vi "Top Level State Machine - Framework Only (working without scripting VIs).vi"() -> ()   [LabVIEW 2014]
uses:
  Scripting States.ctl
  System.Windows.Forms
panel:
  out "Elapsed Time":dbl format="%<%H:%M:%S>t"
  in  "ProgressBar":refnum<k24>(container)
  out "Progress Bar 2":u8
  in  "?":T1
  out "Status Log":string
  out "Progress Bar":u8(slide) scale=0.0..9.0
  # "#TestingOnly"
  # "Append string with new steps as they're reached\nAppend error with source information (including current state) to end if it occurs"
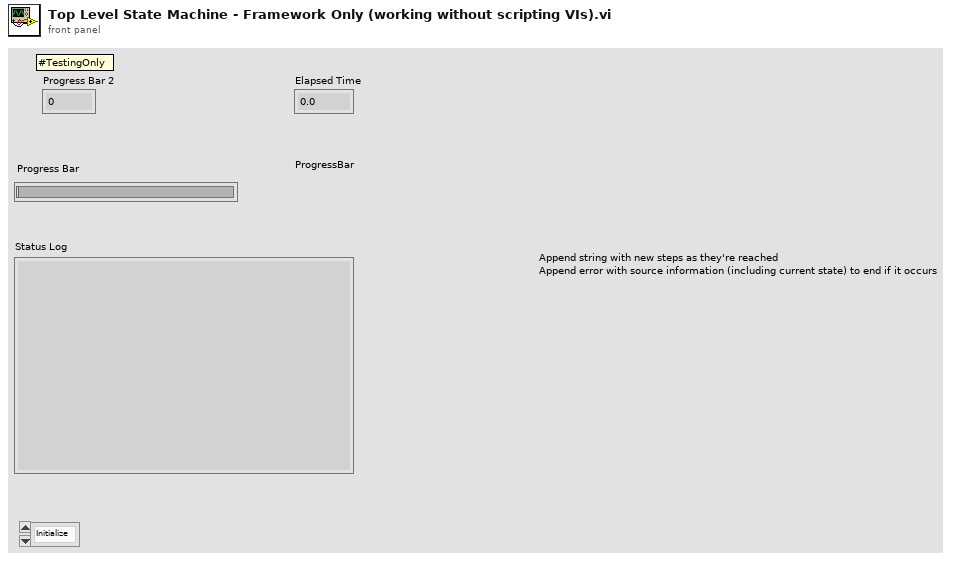
[diagram p1: front panel]
types:
  T1 = typedef "Scripting States.ctl" = enum16{"Initialize", "Modify Dequeue Commands", "Modify Enqueue Data", "Create Project FIFOs", "Populate FIFO Names in Engine", "Create and Place IO Nodes", "Place SPI Engine", "Modify I/O Pin Names", "Modify I/O Pin Enable", "End"}
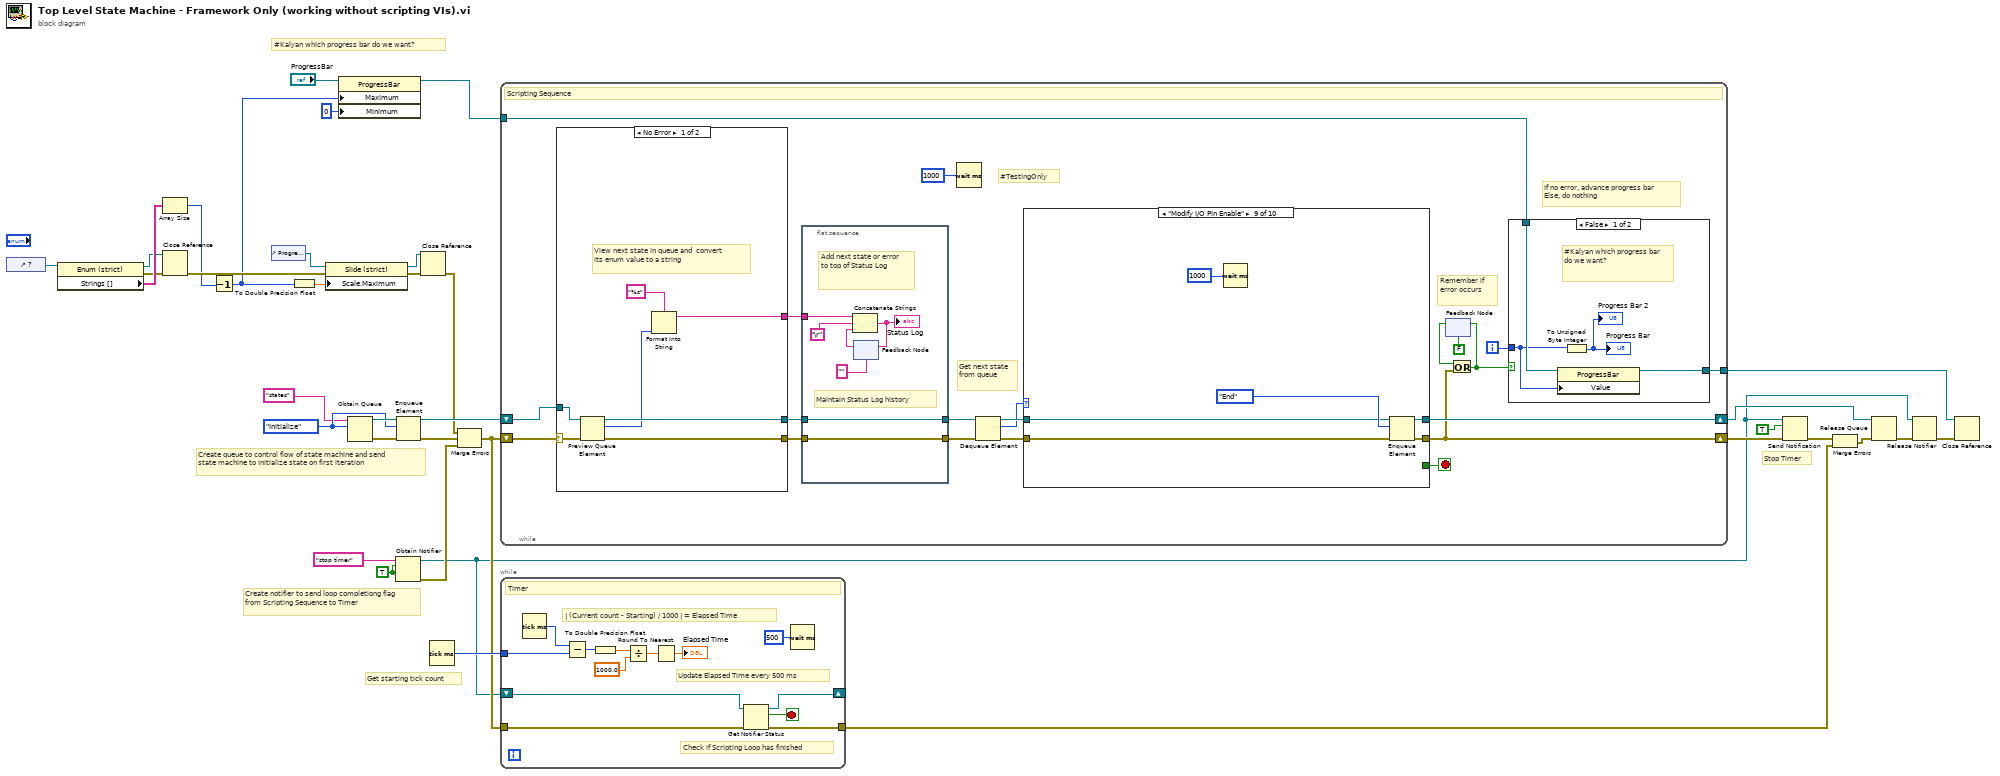
[diagram p0: block diagram]
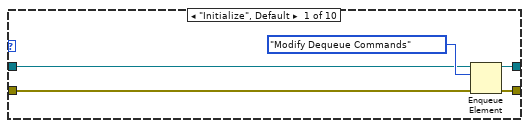
[diagram p3: hidden frame]
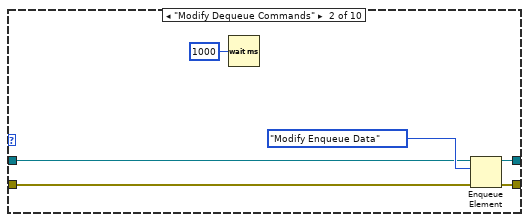
[diagram p4: hidden frame]
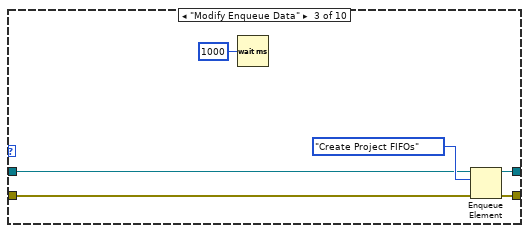
[diagram p5: hidden frame]
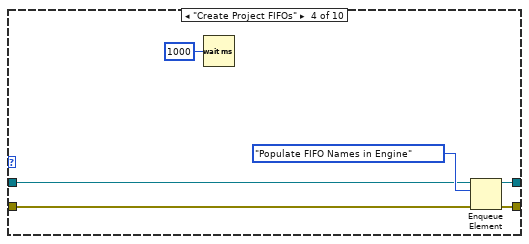
[diagram p6: hidden frame]
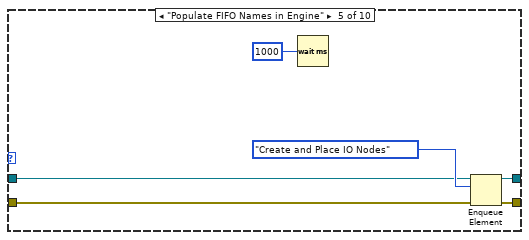
[diagram p7: hidden frame]
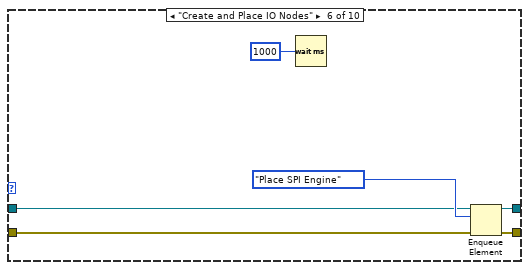
[diagram p8: hidden frame]
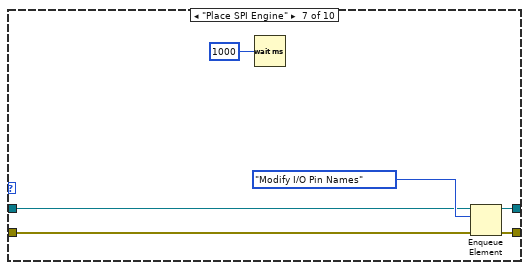
[diagram p9: hidden frame]
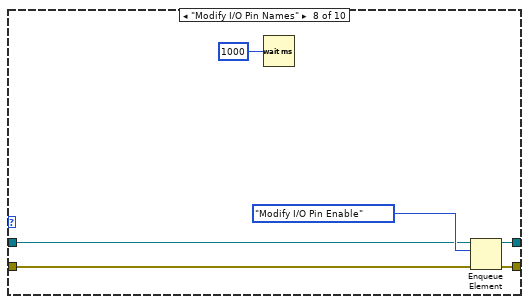
[diagram p10: hidden frame]
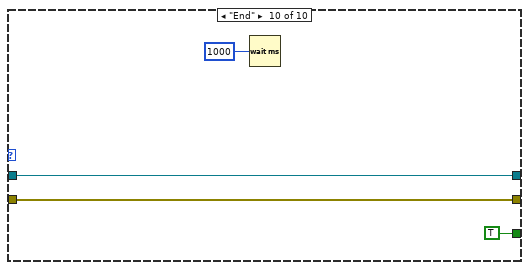
[diagram p11: hidden frame]
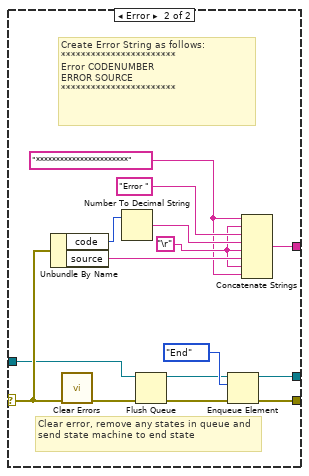
[diagram p12: hidden frame]
diagram:
  w13 = TRUE ("create if not found? (T)")
  w30 = Scripting_States."Initialize"
  # "Get starting tick count"
  # "Stop Timer"
  # "Create notifier to send loop completiong flag from Scripting Sequence to Timer"
  # "Create queue to control flow of state machine and send state machine to Initialize state on first iteration"
  # "#Kalyan which progress bar do we want?"
  n1 = control-ref of="?"() -> (w36:refnum<vi>)
  n2 = property on="Property Node" class="Enum (strict)"(reference=w36) -> (reference out=w23:refnum<vi>, error out=w24:errorcluster, "Strings []"=w35:string[])  [unwired: 1 in]
  n3 = Array Size(array=w35) -> (size(s)=w20:i32)
  n4 = Close Reference(reference=w23, error in (no error)=w24) -> (error out=w21:errorcluster)
  n5 = Decrement(x=w20) -> (x-1=w18:i32)
  n6 = control-ref of="Progress Bar"() -> (w34:refnum<vi>)
  n7 = To Double Precision Float(number=w18) -> (double precision float=w33:dbl)
  n8 = property on="Property Node" class="Slide (strict)"(reference=w34, error in=w21, "Scale.Maximum"=w33) -> (reference out=w25:refnum<vi>, error out=w26:errorcluster)
  n9 = property class="ProgressBar"(reference="ProgressBar", "Maximum"=w18, "Minimum"=0) -> (reference out=w8:refnum<k24>)  [unwired: 1 in, 1 out]
  n10 = Obtain Queue(name (unnamed)="states", element data type=w30) -> (queue out=w31:refnum<queue>, error out=w32:errorcluster)  [unwired: 3 in, 1 out]
  n11 = Obtain Notifier(name (unnamed)="stop timer", notification data type=w13, create if not found? (T)=w13) -> (notifier out=w1:refnum<notifier>, error out=w15:errorcluster)  [unwired: 1 in, 1 out]
  n12 = Enqueue Element(queue=w31, element=w30, error in (no error)=w32) -> (queue out=w28:refnum<queue>, error out=w27:errorcluster)  [unwired: 1 in, 1 out]
  n13 = Close Reference(reference=w25, error in (no error)=w26) -> (error out=w22:errorcluster)
  n14 = Tick Count (ms)() -> (millisecond timer value=w16:u32)
  n15 = Merge Errors(w22, w27, w15) -> (w14:errorcluster)
  n16 = while {
    shift-right: [w48] -> w3
    shift-left: w14 -> [w56]
    shift-right: [w50] -> w2
    shift-left: w28 -> [w55]
    tunnel: [w38] -> w9
    tunnel: w8 -> [w37]
    i -> [w49]
    stop <- w51 stop-if-true
    # "If no error, advance progress bar\nElse, do nothing"
    # "Remember if error occurs"
    # "Get next state from queue"
    # "#TestingOnly"
    # "Scripting Sequence"
    n17 = case shown="No Error" w56 {
      selector: w56 -> [w132 w142]
      tunnel: [w126 w144] -> w43
      tunnel: w55 -> [w131 w137]
      tunnel: [w129 w141] -> w42
      tunnel: [w130 w140] -> w40
      frame No Error {
        # "View next state in queue and  convert its enum value to a string"
        n18 = Preview Queue Element(queue=w131, error in (no error)=w132) -> (queue out=w130:refnum<queue>, element=w127:T1, error out=w129:errorcluster)  [unwired: 1 in, 1 out]
        n19 = Format Into String "Format Into String"(format string="%s", w127) -> (resulting string=w126:string)  [unwired: 2 in, 1 out]
      }
      frame Error {
        w133 = "***********************" ("string")
        w134 = "\r"
        # "Create Error String as follows:\n***********************\nError CODENUMBER\nERROR SOURCE\n***********************"
        # "Clear error, remove any states in queue and send state machine to end state"
        n20 = Unbundle By Name(w142) -> ("code"=w145:i32, "source"=w147:string)
        n21 = call <vilib>:"Clear Errors.vi"("error in (no error)"=w142) -> ("error out"=w139:errorcluster)  [unwired: 5 in, 1 out]
        n22 = Number To Decimal String(number=w145) -> (decimal integer string=w146:string)  [unwired: 1 in]
        n23 = Flush Queue(queue=w137, error in (no error)=w139) -> (queue out=w136:refnum<queue>, error out=w138:errorcluster)  [unwired: 1 out]
        n24 = Enqueue Element(queue=w136, element=Scripting_States."End", error in (no error)=w138) -> (queue out=w140:refnum<queue>, error out=w141:errorcluster)  [unwired: 1 in, 1 out]
        n25 = Concatenate Strings(w133, w134, "Error " ("string"), w146, w134, w147, w134, w133) -> (w144:string)
      }
    }
    n26 = flat-sequence {
      tunnel: w43 -> [w59]
      tunnel: w42 -> [w58]
      tunnel: [w58] -> w41
      tunnel: [w57] -> w39
      tunnel: w40 -> [w57]
      frame #0 {
        # "Maintain Status Log history"
        # "Add next state or error to top of Status Log"
        n27 = feedback #1("") -> (w61:string)
        n28 = Concatenate Strings(w59, "\r", w61) -> (w62:string)
        "Status Log" <- w62
        n29 = feedback-in #1(w62) -> ()
      }
    }
    n30 = Wait (ms)(milliseconds to wait=u32 1000) -> ()  [unwired: 1 out]
    n31 = Dequeue Element(queue=w39, error in (no error)=w41) -> (queue out=w53:refnum<queue>, element=w52:T1, error out=w54:errorcluster)  [unwired: 1 in, 1 out]
    n32 = case shown="\"Modify I/O Pin Enable\"" w52 {
      tunnel: [w72 w78 w84 w90 w96 w102 w108 w114 w120 w122] -> w48
      tunnel: [w73 w79 w85 w91 w97 w103 w109 w115 w121 w124] -> w50
      tunnel: [_ _ _ _ _ _ _ _ _ TRUE] -> w51
      tunnel: w54 -> [w70 w75 w81 w86 w93 w99 w105 w111 w117 w122]
      tunnel: w53 -> [w69 w76 w82 w88 w94 w100 w106 w112 w118 w124]
      frame "Initialize", Default {
        n33 = Enqueue Element(queue=w69, element=Scripting_States."Modify Dequeue Commands", error in (no error)=w70) -> (queue out=w73:refnum<queue>, error out=w72:errorcluster)  [unwired: 1 in, 1 out]
      }
      frame "Modify Dequeue Commands" {
        n34 = Wait (ms)(milliseconds to wait=u32 1000) -> ()  [unwired: 1 out]
        n35 = Enqueue Element(queue=w76, element=Scripting_States."Modify Enqueue Data", error in (no error)=w75) -> (queue out=w79:refnum<queue>, error out=w78:errorcluster)  [unwired: 1 in, 1 out]
      }
      frame "Modify Enqueue Data" {
        n36 = Wait (ms)(milliseconds to wait=u32 1000) -> ()  [unwired: 1 out]
        n37 = Enqueue Element(queue=w82, element=Scripting_States."Create Project FIFOs", error in (no error)=w81) -> (queue out=w85:refnum<queue>, error out=w84:errorcluster)  [unwired: 1 in, 1 out]
      }
      frame "Create Project FIFOs" {
        n38 = Wait (ms)(milliseconds to wait=u32 1000) -> ()  [unwired: 1 out]
        n39 = Enqueue Element(queue=w88, element=Scripting_States."Populate FIFO Names in Engine", error in (no error)=w86) -> (queue out=w91:refnum<queue>, error out=w90:errorcluster)  [unwired: 1 in, 1 out]
      }
      frame "Populate FIFO Names in Engine" {
        n40 = Wait (ms)(milliseconds to wait=u32 1000) -> ()  [unwired: 1 out]
        n41 = Enqueue Element(queue=w94, element=Scripting_States."Create and Place IO Nodes", error in (no error)=w93) -> (queue out=w97:refnum<queue>, error out=w96:errorcluster)  [unwired: 1 in, 1 out]
      }
      frame "Create and Place IO Nodes" {
        n42 = Wait (ms)(milliseconds to wait=u32 1000) -> ()  [unwired: 1 out]
        n43 = Enqueue Element(queue=w100, element=Scripting_States."Place SPI Engine", error in (no error)=w99) -> (queue out=w103:refnum<queue>, error out=w102:errorcluster)  [unwired: 1 in, 1 out]
      }
      frame "Place SPI Engine" {
        n44 = Wait (ms)(milliseconds to wait=u32 1000) -> ()  [unwired: 1 out]
        n45 = Enqueue Element(queue=w106, element=Scripting_States."Modify I/O Pin Names", error in (no error)=w105) -> (queue out=w109:refnum<queue>, error out=w108:errorcluster)  [unwired: 1 in, 1 out]
      }
      frame "Modify I/O Pin Names" {
        n46 = Wait (ms)(milliseconds to wait=u32 1000) -> ()  [unwired: 1 out]
        n47 = Enqueue Element(queue=w112, element=Scripting_States."Modify I/O Pin Enable", error in (no error)=w111) -> (queue out=w115:refnum<queue>, error out=w114:errorcluster)  [unwired: 1 in, 1 out]
      }
      frame "Modify I/O Pin Enable" {
        n48 = Wait (ms)(milliseconds to wait=u32 1000) -> ()  [unwired: 1 out]
        n49 = Enqueue Element(queue=w118, element=Scripting_States."End", error in (no error)=w117) -> (queue out=w121:refnum<queue>, error out=w120:errorcluster)  [unwired: 1 in, 1 out]
      }
      frame "End" {
        n50 = Wait (ms)(milliseconds to wait=u32 1000) -> ()  [unwired: 1 out]
      }
    }
    n51 = feedback #2(FALSE) -> (w47:bool)
    n52 = Or(x=w47, y=w48) -> (x .or. y?=w45:bool)
    n53 = feedback-in #2(w45) -> ()
    n54 = case shown="False" w45 {
      tunnel: w49 -> [w65 _]
      tunnel: [w67 w68] -> w38
      tunnel: w37 -> [w66 w68]
      frame False {
        # "#Kalyan which progress bar do we want?"
        n55 = property class="ProgressBar"(reference=w66, "Value"=w65) -> (reference out=w67:refnum<k24>)  [unwired: 1 in, 1 out]
        n56 = To Unsigned Byte Integer(number=w65) -> (unsigned 8bit integer=→"Progress Bar" →"Progress Bar 2":u8)
      }
      frame True {
      }
    }
  }
  n57 = while {
    tunnel: w16 -> [w159]
    tunnel: w14 -> [w151]
    shift-right: [w149] -> _
    shift-left: w1 -> [w152]
    tunnel: [w148] -> w6
    stop <- w150 stop-if-true
    # "Update Elapsed Time every 500 ms"
    # "| (Current count - Starting) / 1000 | = Elapsed Time"
    # "Check if Scripting Loop has finished"
    # "Timer"
    n58 = Tick Count (ms)() -> (millisecond timer value=w160:u32)
    n59 = Subtract(x=w160, y=w159) -> (x-y=w158:u32)
    n60 = To Double Precision Float(number=w158) -> (double precision float=w157:dbl)
    n61 = Divide(x=w157, y=1000.0) -> (x/y=w155:dbl)
    n62 = Round To Nearest(number=w155) -> (nearest integer value=→"Elapsed Time":dbl)
    n63 = Get Notifier Status(notifier=w152, error in (no error)=w151) -> (notifier out=w149:refnum<notifier>, current notification=w150:bool, error out=w148:errorcluster)  [unwired: 2 out]
    n64 = Wait (ms)(milliseconds to wait=u32 500) -> ()  [unwired: 1 out]
  }
  n65 = Send Notification(notification=TRUE, notifier=w1, error in (no error)=w3) -> (error out=w4:errorcluster)  [unwired: 1 out]
  n66 = Merge Errors(w4, w6) -> (w7:errorcluster)
  n67 = Release Queue(queue=w2, error in (no error)=w7) -> (error out=w11:errorcluster)  [unwired: 1 in, 2 out]
  n68 = Release Notifier(notifier=w1, error in (no error)=w11) -> (error out=w10:errorcluster)  [unwired: 1 in, 2 out]
  n69 = Close Reference(reference=w9, error in (no error)=w10) -> ()  [unwired: 1 out]
